vi "Create Field Object.vi"(8 "error in (no error)":errorcluster, 9 "FieldWidthY":i32, 10 "FieldLengthX":i32, 11 "Field in":refnum<class "Field.lvclass">) -> (0 "error out":errorcluster, 3 "Field out":refnum<class "Field.lvclass">)   [LabVIEW 2014, in "Field.lvclass"]
uses:
  Field.lvclass
  Field.lvclass/Field.ctl
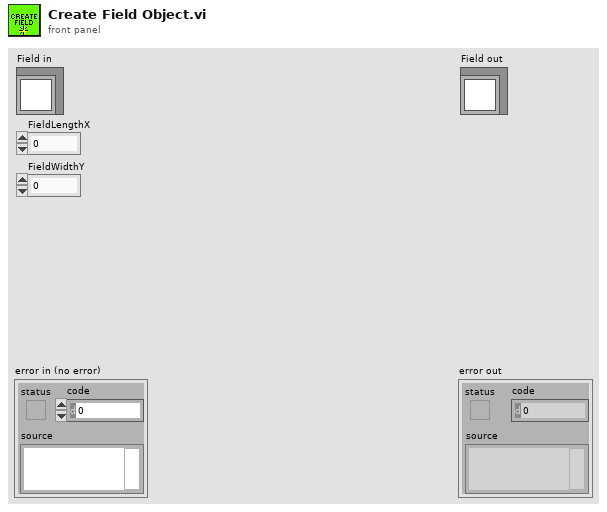
[diagram p1: front panel]
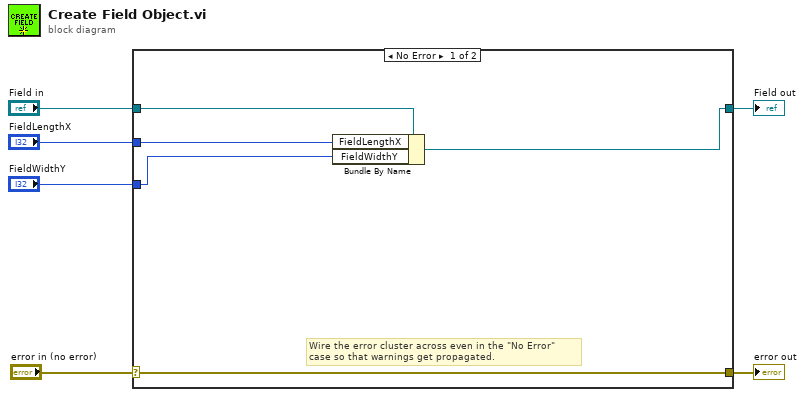
[diagram p0: block diagram]
diagram:
  n1 = case shown="No Error" "error in (no error)" {
    selector: "error in (no error)" -> [w11 w13]
    tunnel: [w11 w13] -> w5
    tunnel: [w7 w12] -> w3
    tunnel: "Field in" -> [w8 w12]
    tunnel: "FieldLengthX" -> [w10 _]
    tunnel: "FieldWidthY" -> [w9 _]
    frame No Error {
      # "Wire the error cluster across even in the \"No Error\"\ncase so that warnings get propagated."
      n2 = Bundle By Name(cluster=w8, "FieldLengthX"=w10, "FieldWidthY"=w9) -> (w7:refnum<class "Field.lvclass">)
    }
    frame Error {
    }
  }
  "error out" <- w5
  "Field out" <- w3
